vi "stop.search.vi"(8 "error in (no error)":errorcluster, 11 "comic_crawler in":refnum<class "comic_crawler.lvclass">) -> (0 "error out":errorcluster, 3 "comic_crawler out":refnum<class "comic_crawler.lvclass">)   [LabVIEW 2024, in "comic_crawler.lvclass"]
uses:
  comic_crawler.lvclass
  daemon.states--enum.ctl
  comic_crawler.lvclass/comic_crawler.ctl
  WebScraper/comic_class/comic_class.lvclass
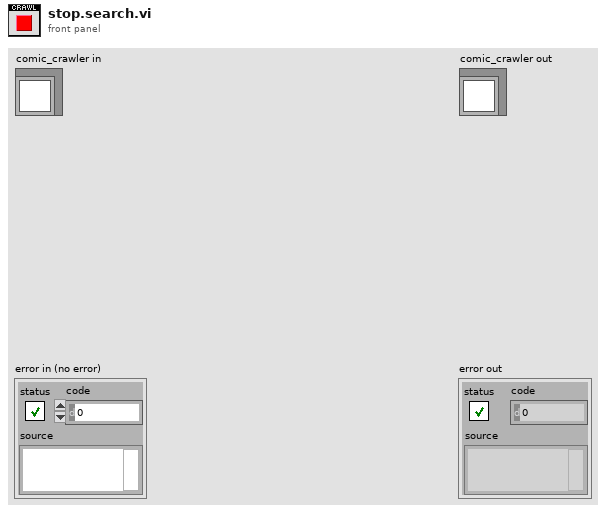
[diagram p1: front panel]
types:
  T1 = typedef "comic_crawler.lvclass/daemon.states--enum.ctl" = enum16{"start search", "idle", "set timer", "running", "stop search", "wait", "set delay", "shut down"}
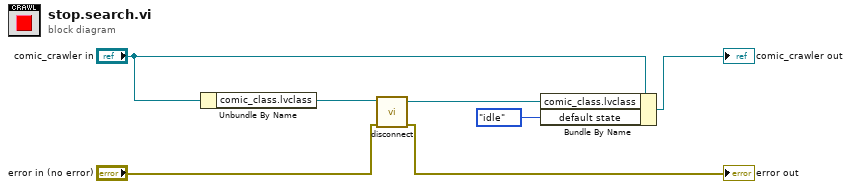
[diagram p0: block diagram]
diagram:
  n1 = Unbundle By Name("comic_crawler in") -> ("comic_class.lvclass"=w7:refnum<class "comic_class.lvclass">)
  n2 = call-dynamic "disconnect.vi"("error in (no error)"="error in (no error)", "comic_class in"=w7) -> ("error out"=→"error out":errorcluster, "comic_class out"=w3:refnum<class "comic_class.lvclass">)  [unwired: 8 in]
  n3 = Bundle By Name(cluster="comic_crawler in", "comic_class.lvclass"=w3, "default state"=daemon.states--enum."idle" ("cmd")) -> (→"comic_crawler out":refnum<class "comic_crawler.lvclass">)
